vi "DAQ.vi"   [LabVIEW 2017, in "DAQ.lvlib"]
uses:
  DAQ.lvlib
  Communication/Communication.lvlib
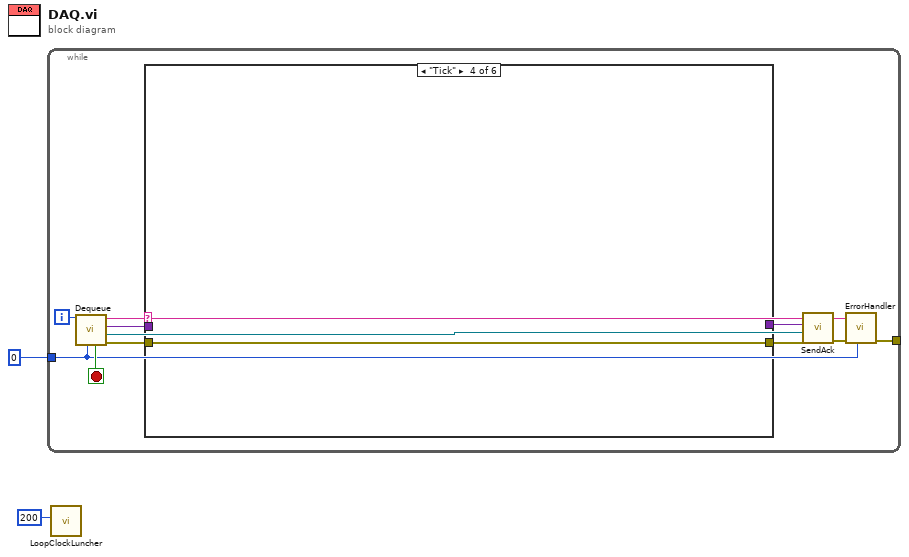
[diagram p0: block diagram]
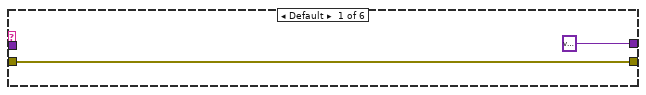
[diagram p2: hidden frame]
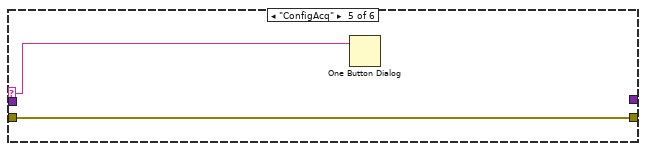
[diagram p5: hidden frame]
diagram:
  n1 = while {
    tunnel: 0 -> [w5]
    tunnel: [w7] -> _
    i -> [w6]
    stop <- w13 stop-if-true
    n2 = call "Dequeue.vi"("Instance"=w5, "Loop Counter"=w6) -> ("error out"=w10:errorcluster, "ResponseNotifcation"=w11:refnum<notifier>, "Data"=w12:variant, "Msg"=w4:string, "Exit?"=w13:bool)  [unwired: 5 in]
    n3 = case shown="\"Tick\"" w4 {
      selector: w4 -> [_ _ _ _ w19 _]
      tunnel: w12 -> [_ _ _ _ _ _]
      tunnel: w10 -> [w15 w16 w17 w18 w20 w21]
      tunnel: [variant _ _ _ _ _] -> w9
      tunnel: [w15 w16 w17 w18 w20 w21] -> w3
      frame Default {
      }
      frame "Init" {
      }
      frame "Exit" {
      }
      frame "Tick" {
      }
      frame "ConfigAcq" {
        n4 = One Button Dialog(message=w19) -> ()  [unwired: 1 in, 1 out]
      }
      frame "Error" {
      }
    }
    n5 = call "SendAck.vi"("error in (no error)"=w3, "Ack"=w11, "Variant"=w9) -> ("error out"=w8:errorcluster)  [unwired: 8 in]
    n6 = call "ErrorHandler.vi"("Instance"=w5, "error in (no error)"=w8, "Msg"=w4) -> ("error out"=w7:errorcluster)  [unwired: 8 in]
  }
  n7 = call "LoopClockLuncher.vi"("milliseconds to wait"=200) -> ()  [unwired: 9 in, 2 out]
